vi "GetType.vi"(8 "error in (no error)":errorcluster, 11 "Mute Single Msg":refnum<class "Mute Single Msg.lvclass">) -> (0 "error out":errorcluster, 2 "Data Sample":variant, 3 "Mute Single Msg":refnum<class "Mute Single Msg.lvclass">)   [LabVIEW 2016, in "KIT-QVA.lvlib" / "Mute Single Msg.lvclass"]
doc: "This VI delivers a sample of the data type format the message expects."
uses:
  Mute Single Msg.lvclass
  Mute Single Msg.lvclass/Mute Single Msg.ctl
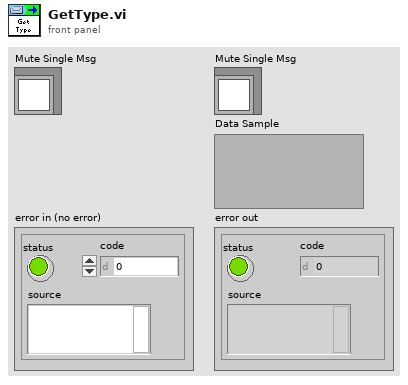
[diagram p1: front panel]
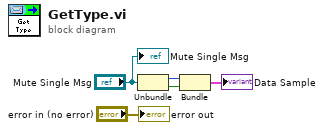
[diagram p0: block diagram]
diagram:
  n1 = Unbundle("Mute Single Msg") -> (w2:u8, w1:bool)
  n2 = Bundle("Detector"=w2, "Mute"=w1) -> (→"Data Sample":cluster{"Detector":u8, "Mute":bool})  [unwired: 1 in]
  "error out" <- "error in (no error)"
  "Mute Single Msg" <- "Mute Single Msg"
